vi "Clear Data.vi"(8 "error in (no error)":errorcluster, 11 "MCLB_Lib in":refnum<class "MCLB_Lib.lvclass">) -> (0 "error out":errorcluster, 3 "MCLB_Lib out":refnum<class "MCLB_Lib.lvclass">)   [LabVIEW 2020, in "MCLB_Lib.lvclass"]
uses:
  MCLB_Lib.lvclass
  MCLB_Lib.lvclass/MCLB_Lib.ctl
  <vilib>/Utility/miscctls.llb/LVRowAndColumnUnsignedTypeDef.ctl
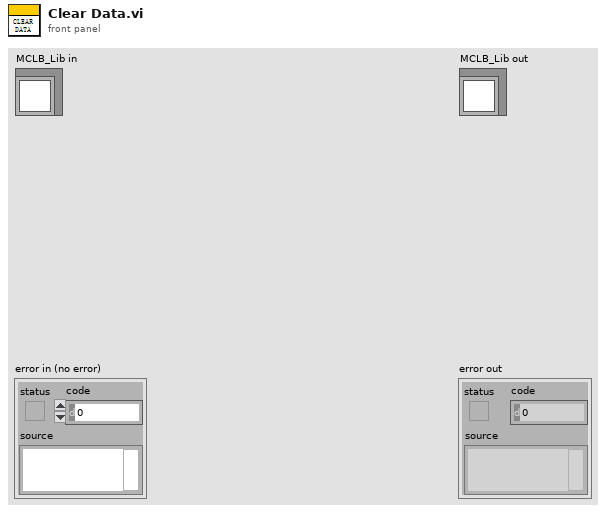
[diagram p1: front panel]
types:
  T1 = typedef "LVRowAndColumnUnsignedTypeDef.ctl" = cluster{"Row":u32, "Column":u32}
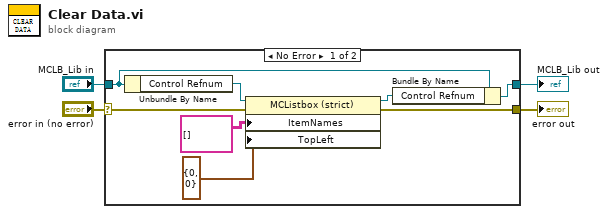
[diagram p0: block diagram]
diagram:
  n1 = case shown="No Error" "error in (no error)" {
    selector: "error in (no error)" -> [w8 w14]
    tunnel: [w7 w14] -> w3
    tunnel: [w10 w13] -> w1
    tunnel: "MCLB_Lib in" -> [w12 w13]
    frame No Error {
      n2 = Unbundle By Name(w12) -> ("Control Refnum"=w11:refnum<vi>)
      n3 = property class="MCListbox (strict)"(reference=w11, error in=w8, "ItemNames"=string[][] [] ("Item Names"), "TopLeft"=T1 {"Row"=0, "Column"=0} ("Top Left Visible Cell")) -> (reference out=w9:refnum<vi>, error out=w7:errorcluster)
      n4 = Bundle By Name(cluster=w12, "Control Refnum"=w9) -> (w10:refnum<class "MCLB_Lib.lvclass">)
    }
    frame Error {
    }
  }
  "error out" <- w3
  "MCLB_Lib out" <- w1
